vi "Two Bodies.vi"(7 "Data":T1) -> (0 "Simulation Objects":refnum<class "SimulationObject.lvclass">[](array[class]), 1 "Cell Size":i16, 2 "Gravity Vector out":refnum<class "Vector2.lvclass">, 3 "Background Color out":u32(colorbox))   [LabVIEW 2022 SP3]
uses:
  Engine/Math/Vector2/Vector2.lvclass
  Engine/Objects/SimulationObject/SimulationObject.lvclass
  Engine/Math/Vector2/Vector2.lvclass/Vector2.ctl
  Engine/Objects/SimulationObject/SimulationObject.lvclass/SimulationObject.ctl
  Engine/Objects/Components/PhysicsComponent/PhysicsComponent.lvclass/PhysicsComponent.ctl
  Engine/Objects/Shapes/CircleShape/CircleShape.lvclass
  D:/Programowanie/Studia/Labview/CollisionSimulator/Project/Engine/Objects/Shapes/Shapeable/Shapeable.lvclass
  Engine/Objects/Components/PhysicsComponent/PhysicsComponent.lvclass
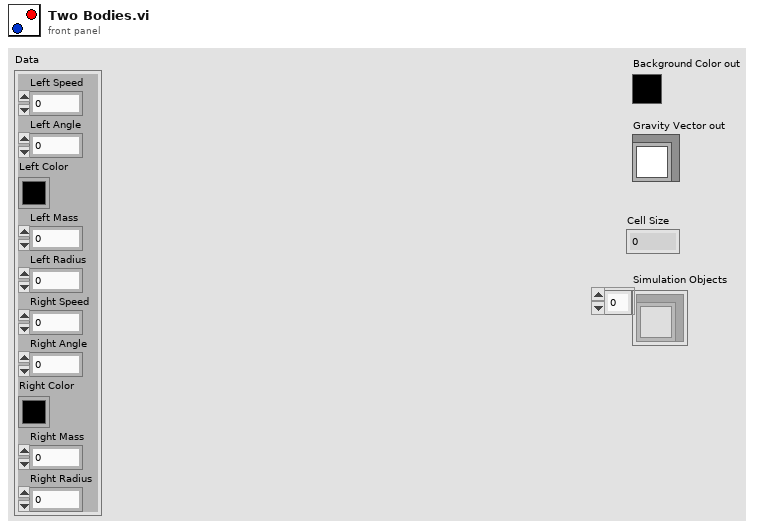
[diagram p1: front panel]
types:
  T1 = cluster{"Left Speed":dbl, "Left Angle":dbl, "Left Color":u32, "Left Mass":dbl, "Left Radius":dbl, "Right Speed":dbl, "Right Angle":dbl, "Right Color":u32, "Right Mass":dbl, "Right Radius":dbl}
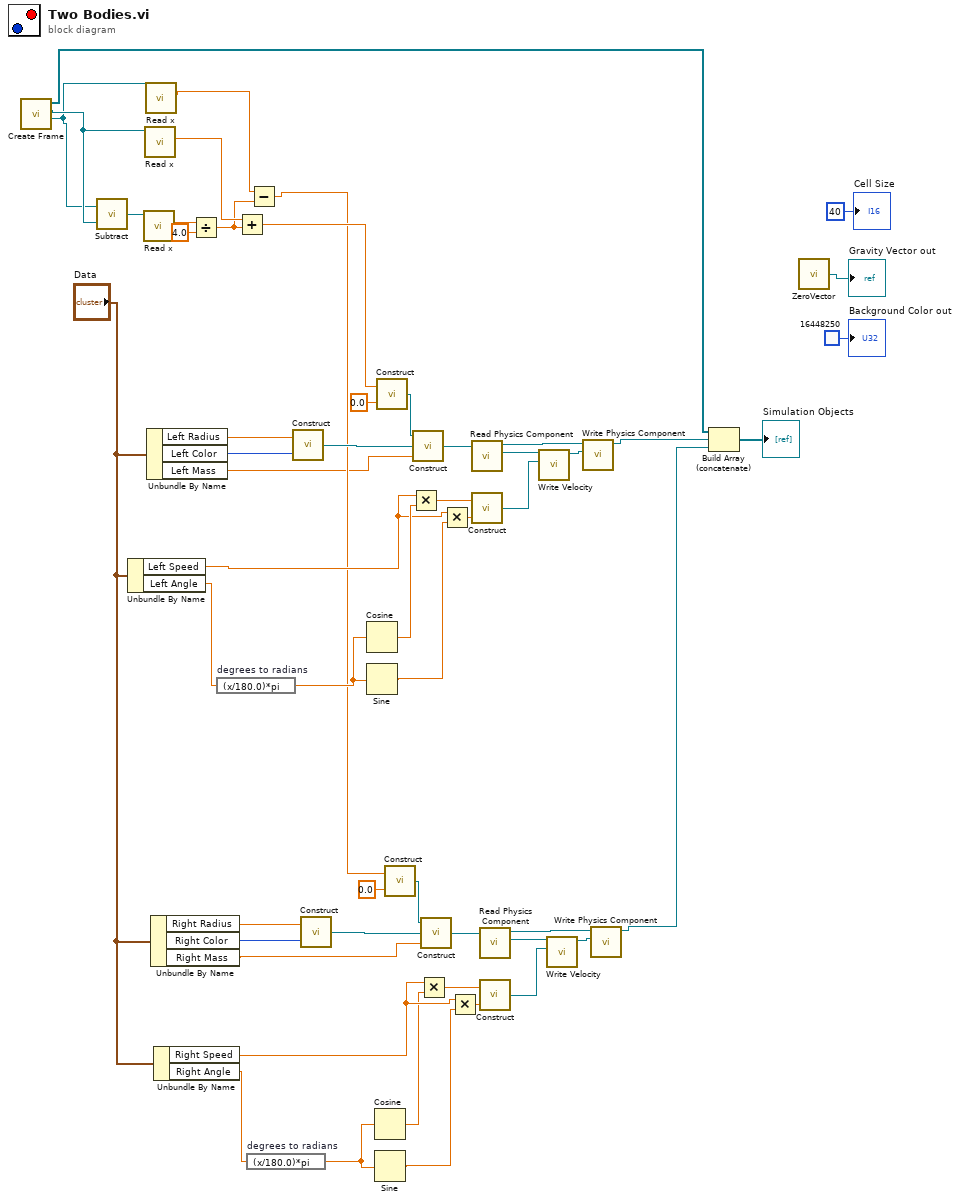
[diagram p0: block diagram]
diagram:
  n1 = call "Create Frame.vi"() -> ("Max Available Position"=w11:refnum<class "Vector2.lvclass">, "Min Available Position"=w33:refnum<class "Vector2.lvclass">, "Simulation Objects"=w4:refnum<class "SimulationObject.lvclass">[])  [unwired: 4 in, 1 out]
  n2 = call "Subtract.vi"("Vec2 b in"=w33, "Vec2 a in"=w11) -> ("Vec2 out"=w34:refnum<class "Vector2.lvclass">)
  n3 = Unbundle By Name("Data") -> ("Left Speed"=w35:dbl, "Left Angle"=w41:dbl)
  n4 = call "Read x.vi"("Vector2 in"=w34) -> ("x"=w32:sgl)  [unwired: 8 in, 2 out]
  n5 = call "Read x.vi"("Vector2 in"=w33) -> ("x"=w30:sgl)  [unwired: 8 in, 2 out]
  n6 = call "Read x.vi"("Vector2 in"=w11) -> ("x"=w10:sgl)  [unwired: 8 in, 2 out]
  n7 = Unbundle By Name("Data") -> ("Left Radius"=w42:dbl, "Left Color"=w43:u32, "Left Mass"=w5:dbl)
  n8 = Unbundle By Name("Data") -> ("Right Radius"=w21:dbl, "Right Color"=w20:u32, "Right Mass"=w6:dbl)
  n9 = Unbundle By Name("Data") -> ("Right Speed"=w28:dbl, "Right Angle"=w22:dbl)
  n10 = Divide(x=w32, y=sgl 4.0) -> (x/y=w9:sgl)
  n11 = expression code="(x/180.0)*pi" "degrees to radians"(w41) -> (w40:dbl)
  n12 = Add(x=w30, y=w9) -> (x+y=w29:sgl)
  n13 = expression code="(x/180.0)*pi" "degrees to radians"(w22) -> (w23:dbl)
  n14 = Subtract(x=w10, y=w9) -> (x-y=w8:sgl)
  n15 = call "Construct.vi"("Color"=w43, "Radius"=w42) -> ("CircleShape out"=w47:refnum<class "CircleShape.lvclass">)
  n16 = call "Construct.vi"("Color"=w20, "Radius"=w21) -> ("CircleShape out"=w19:refnum<class "CircleShape.lvclass">)
  n17 = Cosine(x=w40) -> (cos(x)=w37:dbl)
  n18 = Sine(x=w40) -> (sin(x)=w36:dbl)
  n19 = Cosine(x=w23) -> (cos(x)=w26:dbl)
  n20 = Sine(x=w23) -> (sin(x)=w27:dbl)
  n21 = call "Construct.vi"("y"=sgl 0.0, "x"=w29) -> ("Vec2 out"=w49:refnum<class "Vector2.lvclass">)
  n22 = call "Construct.vi"("y"=sgl 0.0, "x"=w8) -> ("Vec2 out"=w17:refnum<class "Vector2.lvclass">)
  n23 = Multiply(x=w35, y=w37) -> (x*y=w39:dbl)
  n24 = call "Construct.vi"("Mass"=w5, "Shape in"=w47, "Local Position in"=w49) -> ("Simulation Object out"=w50:refnum<class "SimulationObject.lvclass">)
  n25 = Multiply(x=w28, y=w26) -> (x*y=w24:dbl)
  n26 = call "Construct.vi"("Mass"=w6, "Shape in"=w19, "Local Position in"=w17) -> ("Simulation Object out"=w16:refnum<class "SimulationObject.lvclass">)
  n27 = Multiply(x=w35, y=w36) -> (x*y=w38:dbl)
  n28 = Multiply(x=w28, y=w27) -> (x*y=w25:dbl)
  n29 = call "Read Physics Component.vi"("SimulationObject in"=w50) -> ("Physics Component out"=w53:refnum<class "PhysicsComponent.lvclass">, "SimulationObject out"=w51:refnum<class "SimulationObject.lvclass">)  [unwired: 8 in, 1 out]
  n30 = call "Construct.vi"("y"=w38, "x"=w39) -> ("Vec2 out"=w54:refnum<class "Vector2.lvclass">)
  n31 = call "Read Physics Component.vi"("SimulationObject in"=w16) -> ("Physics Component out"=w13:refnum<class "PhysicsComponent.lvclass">, "SimulationObject out"=w15:refnum<class "SimulationObject.lvclass">)  [unwired: 8 in, 1 out]
  n32 = call "Construct.vi"("y"=w25, "x"=w24) -> ("Vec2 out"=w12:refnum<class "Vector2.lvclass">)
  n33 = call "Write Velocity.vi"("Velocity in"=w54, "PhysicsComponent in"=w53) -> ("PhysicsComponent out"=w52:refnum<class "PhysicsComponent.lvclass">)  [unwired: 8 in, 1 out]
  n34 = call "Write Velocity.vi"("Velocity in"=w12, "PhysicsComponent in"=w13) -> ("PhysicsComponent out"=w14:refnum<class "PhysicsComponent.lvclass">)  [unwired: 8 in, 1 out]
  n35 = call "Write Physics Component.vi"("PhysicsComponent.lvclass"=w52, "SimulationObject in"=w51) -> ("SimulationObject out"=w3:refnum<class "SimulationObject.lvclass">)  [unwired: 8 in, 1 out]
  n36 = call "Write Physics Component.vi"("PhysicsComponent.lvclass"=w14, "SimulationObject in"=w15) -> ("SimulationObject out"=w2:refnum<class "SimulationObject.lvclass">)  [unwired: 8 in, 1 out]
  n37 = Build Array (concatenate)(w4, w3, w2) -> (→"Simulation Objects":refnum<class "SimulationObject.lvclass">[])
  n38 = call "ZeroVector.vi"() -> ("Zero Vector"=→"Gravity Vector out":refnum<class "Vector2.lvclass">)
  "Background Color out" <- u32 16448250 ("Background Color out")
  "Cell Size" <- i16 40 ("Cell Size")
